vi "CheckIfRight&WrongTargetsTouched.vi"(3 "Target":T1(ring), 4 "Touch sensor lines":T2={"Home touch"=3, "Touch 1"=1, "Touch 2"=2, "Touch 3"=4, "Touch 4"=4}, 6 "Home+target OK?":bool, 7 "DI Task":refnum<k21>) -> (0 "Wrong target touched?":bool, 1 "Target touched?":bool)   [LabVIEW 2010]
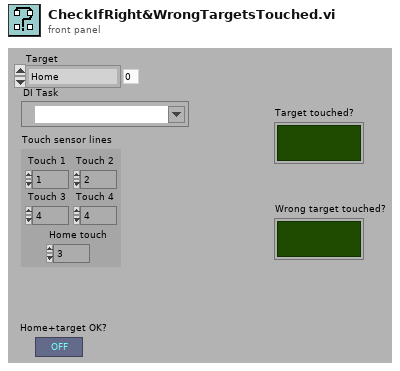
[diagram p1: front panel]
types:
  T1 = enum16{"Home", "Touch 1", "Touch 2", "Touch 3", "Touch 4", "None"}
  T2 = cluster{"Home touch":i16, "Touch 1":i16, "Touch 2":i16, "Touch 3":i16, "Touch 4":i16}
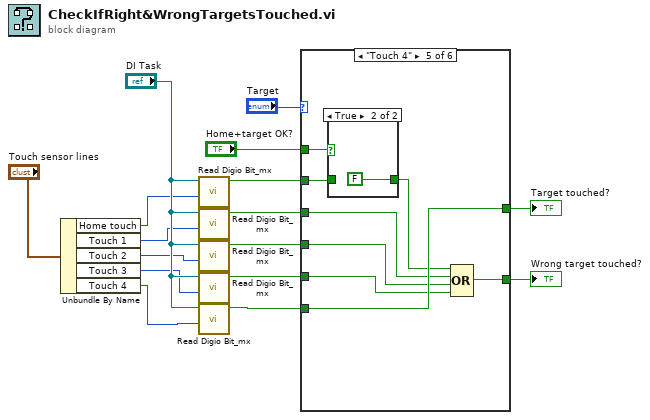
[diagram p0: block diagram]
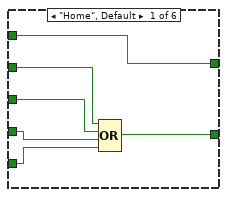
[diagram p2: hidden frame]
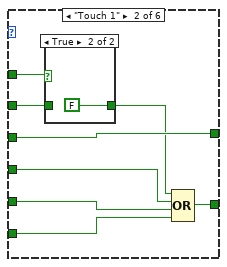
[diagram p3: hidden frame]
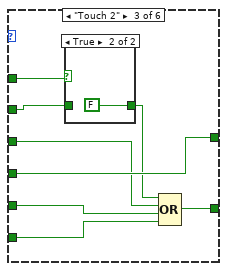
[diagram p5: hidden frame]
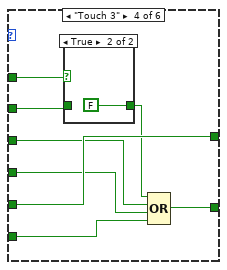
[diagram p7: hidden frame]
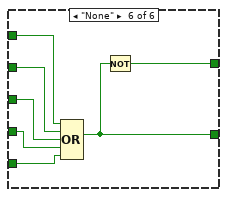
[diagram p10: hidden frame]
diagram:
  n1 = Unbundle By Name("Touch sensor lines") -> ("Home touch"=w10:i16, "Touch 1"=w9:i16, "Touch 2"=w8:i16, "Touch 3"=w7:i16, "Touch 4"=w6:i16)
  n2 = call "Read Digio Bit_mx.vi"("line"=w10, "DI Task"="DI Task") -> ("line state"=w1:bool)  [unwired: 7 in, 1 out]
  n3 = call "Read Digio Bit_mx.vi"("line"=w9, "DI Task"="DI Task") -> ("line state"=w2:bool)  [unwired: 7 in, 1 out]
  n4 = call "Read Digio Bit_mx.vi"("line"=w8, "DI Task"="DI Task") -> ("line state"=w3:bool)  [unwired: 7 in, 1 out]
  n5 = call "Read Digio Bit_mx.vi"("line"=w7, "DI Task"="DI Task") -> ("line state"=w4:bool)  [unwired: 7 in, 1 out]
  n6 = call "Read Digio Bit_mx.vi"("line"=w6, "DI Task"="DI Task") -> ("line state"=w5:bool)  [unwired: 7 in, 1 out]
  n7 = case shown="\"Touch 4\"" "Target" {
    tunnel: w1 -> [w21 w24 w34 w45 w54 w66]
    tunnel: w2 -> [w17 w29 w36 w46 w56 w67]
    tunnel: w3 -> [w18 w26 w39 w47 w57 w68]
    tunnel: w4 -> [w19 w27 w37 w49 w58 w69]
    tunnel: w5 -> [w20 w28 w38 w48 w59 w65]
    tunnel: [w22 w30 w40 w50 w60 w63] -> w15
    tunnel: [w21 w29 w39 w49 w59 w64] -> w16
    tunnel: "Home+target OK?" -> [_ w25 w35 w43 w55 _]
    frame "Home", Default {
      n8 = Compound Arithmetic op=OR(w17, w18, w19, w20) -> (w22:bool)
    }
    frame "Touch 1" {
      n9 = case shown="True" w25 {
        tunnel: [w31 FALSE ("line state")] -> w23
        tunnel: w24 -> [w31 _]
        frame False {
        }
        frame True {
        }
      }
      n10 = Compound Arithmetic op=OR(w23, w26, w27, w28) -> (w30:bool)
    }
    frame "Touch 2" {
      n11 = case shown="True" w35 {
        tunnel: [w41 FALSE ("line state")] -> w33
        tunnel: w34 -> [w41 _]
        frame False {
        }
        frame True {
        }
      }
      n12 = Compound Arithmetic op=OR(w33, w36, w37, w38) -> (w40:bool)
    }
    frame "Touch 3" {
      n13 = case shown="True" w43 {
        tunnel: [w51 FALSE ("line state")] -> w44
        tunnel: w45 -> [w51 _]
        frame False {
        }
        frame True {
        }
      }
      n14 = Compound Arithmetic op=OR(w44, w46, w47, w48) -> (w50:bool)
    }
    frame "Touch 4" {
      n15 = case shown="True" w55 {
        tunnel: [w61 FALSE ("line state")] -> w53
        tunnel: w54 -> [w61 _]
        frame False {
        }
        frame True {
        }
      }
      n16 = Compound Arithmetic op=OR(w53, w56, w57, w58) -> (w60:bool)
    }
    frame "None" {
      n17 = Compound Arithmetic op=OR(w66, w67, w68, w69, w65) -> (w63:bool)
      n18 = Not(x=w63) -> (.not. x?=w64:bool)
    }
  }
  "Target touched?" <- w16
  "Wrong target touched?" <- w15
